vi "_FPGA Check CurGas.vi"(4 "error in":errorcluster, 5 "DisableCheck (F)":bool, 6 "CheckNow (F)":bool) -> (0 "error out":errorcluster, 2 "CurGasOK":bool)   [LabVIEW 2012]
uses:
  Type/_LED States.ctl
  Type/_LCD Line2 Msg.ctl
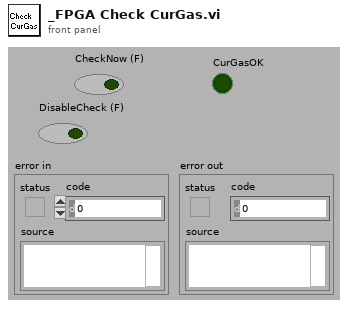
[diagram p1: front panel]
types:
  T1 = typedef "_LED States.ctl" = enum8{"Idle", "Solid B", "Solid R", "Solid P", "Off B", "Off R", "Off P", "Off BRP", "Off RP", "Flash R&P", "Flash P"}
  T2 = typedef "_LCD Line2 Msg.ctl" = u16
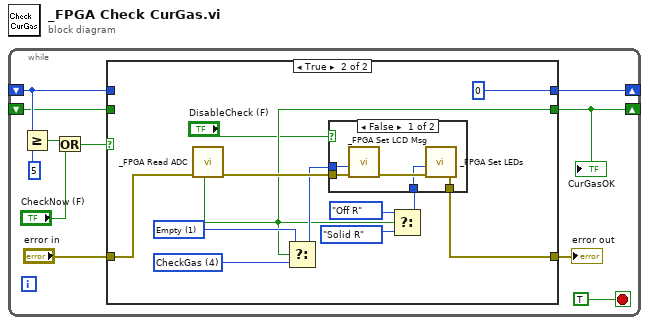
[diagram p0: block diagram]
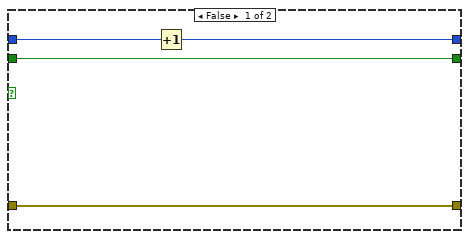
[diagram p2: hidden frame]
diagram:
  n1 = while {
    shift-right: [w10] -> _
    shift-left: _ -> [w5]
    shift-right: [w1] -> _
    shift-left: _ -> [w2]
    stop <- TRUE stop-if-true
    n2 = Greater Or Equal?(x=w5, y=5) -> (x >= y?=w8:bool)
    n3 = Or(x=w8, y="CheckNow (F)") -> (x .or. y?=w6:bool)
    n4 = case shown="True" w6 {
      tunnel: [w14 0] -> w10
      tunnel: w5 -> [w15 _]
      tunnel: [w13 w21] -> w3
      tunnel: "error in" -> [w13 w26]
      tunnel: [w12 w17] -> w1
      tunnel: w2 -> [w12 _]
      frame False {
        n5 = Increment(x=w15) -> (x+1=w14:i32)
      }
      frame True {
        w20 = T2 1 items=["Same", "Empty", "VacFail", "Cancel", "CheckGas", "EleFail", "Probe1Fail", "Probe2Fail", "HeaterFail", "DoorOpen", "CheckComm", "PressStart"] ("Line2Msg (same)")
        w19 = T2 4 items=["Same", "Empty", "VacFail", "Cancel", "CheckGas", "EleFail", "Probe1Fail", "Probe2Fail", "HeaterFail", "DoorOpen", "CheckComm", "PressStart"] ("Line2Msg (same)")
        n6 = call "_FPGA Read ADC.vi"("error in"=w26) -> ("error out"=w25:errorcluster, "In Range?"=w17:bool)  [unwired: 2 in, 5 out]
        n7 = Select(t=w20, s=w17, f=w19) -> (s? t:f=w18:T2)
        n8 = Select(t=_LED_States."Off R" ("LED Command"), s=w17, f=_LED_States."Solid R" ("LED Command")) -> (s? t:f=w22:T1)
        n9 = case shown="False" "DisableCheck (F)" {
          tunnel: w25 -> [w32 w33]
          tunnel: w22 -> [w30 _]
          tunnel: [w29 w33] -> w21
          tunnel: w18 -> [w28 _]
          frame False {
            n10 = call "_FPGA Set LCD Msg.vi"("error in"=w32, "Line2Msg (same)"=w28) -> ("error out"=w31:errorcluster)  [unwired: 5 in, 2 out]
            n11 = call "_FPGA Set LEDs.vi"("error in (no error)"=w31, "LED Command"=w30) -> ("error out"=w29:errorcluster)  [unwired: 2 in, 3 out]
          }
          frame True {
          }
        }
      }
    }
    "error out" <- w3
    "CurGasOK" <- w1
  }
